vi "Get Config Files Directory.vi"() -> (3 "configuration file path":path)   [LabVIEW 2018, in "Configuration File.lvlib" / "Configuration File.lvclass"]
doc: "This VI delivers the directory to search for the configuration files in both the roboRIO and the local machine."
uses:
  Configuration File.lvclass
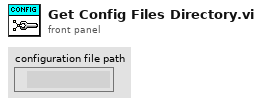
[diagram p1: front panel]
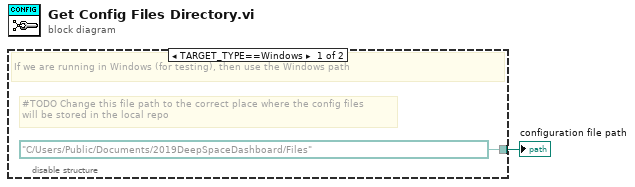
[diagram p0: block diagram]
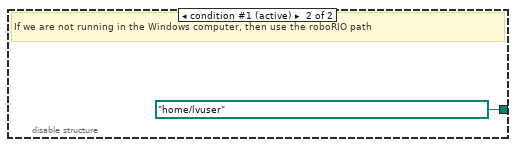
[diagram p2: hidden frame]
diagram:
  n1 = disable-structure shown="TARGET_TYPE==Windows" {
    disable-tunnel: [path "C:/Users/Public/Documents/2019DeepSpaceDashboard/Files" ("configuration file path") path "/home/lvuser" ("configuration file path")] -> w1
    frame condition #0 {
      # "#TODO Change this file path to the correct place where the config files\nwill be stored in the local repo"
      # "If we are running in Windows (for testing), then use the Windows path"
    }
    frame condition #1 (active) {
      # "If we are not running in the Windows computer, then use the roboRIO path"
    }
  }
  "configuration file path" <- w1
